vi "PraksIP.vi"() -> ()   [LabVIEW 2018]
panel:
  out "Received data":string
  in  "remote port or service name":u16
  in  "address":string
  in  "stop":bool
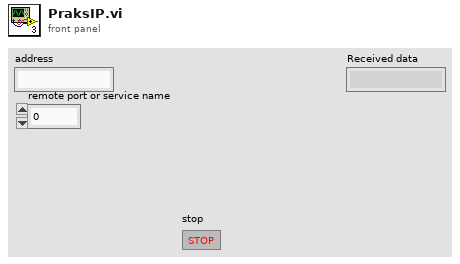
[diagram p1: front panel]
types:
  T1 = enum16{"Standard", "Buffered", "CRLF", "Immediate"}
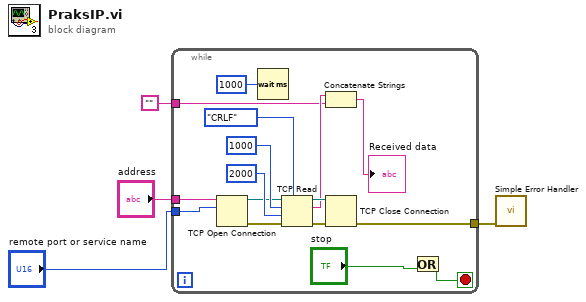
[diagram p0: block diagram]
diagram:
  n1 = while {
    tunnel: "address" -> [w19]
    tunnel: "remote port or service name" -> [w18]
    tunnel: [w10] -> w2
    tunnel: "" -> [w8]
    stop <- w5 stop-if-true
    n2 = TCP Open Connection(address=w19, remote port or service name=w18) -> (connection ID=w14:refnum<k5>, error out=w11:errorcluster)  [unwired: 3 in]
    n3 = Wait (ms)(milliseconds to wait=u32 1000) -> ()  [unwired: 1 out]
    n4 = TCP Read(connection ID=w14, bytes to read=1000, error in (no error)=w11, 7:T1."CRLF" ("mode (standard)"), 9:2000 ("timeout ms (25000)")) -> (connection ID out=w13:refnum<k5>, data out=w9:string, error out=w12:errorcluster)
    n5 = Concatenate Strings(w9, w8) -> (→"Received data":string)
    n6 = TCP Close Connection(connection ID=w13, error in (no error)=w12) -> (error out=w10:errorcluster)  [unwired: 1 in, 1 out]
    n7 = Or(y="stop") -> (x .or. y?=w5:bool)  [unwired: 1 in]
  }
  n8 = call <vilib>:"Simple Error Handler.vi"("error in (no error)"=w2) -> ()  [unwired: 4 in, 5 out]
